vi "gfitsio-check-col-for-read.vi"(6 "row":i32, 8 "error in (no error)":errorcluster, 11 "gfits refnum":T1) -> (0 "error out":errorcluster, 3 "dup gfits refnum":T1)   [LabVIEW 2022 SP3, in "gfitsio.lvlib"]
uses:
  gfitsio.lvlib
  gfitsio-refnum.ctl
  gfitsio-error-codes.ctl
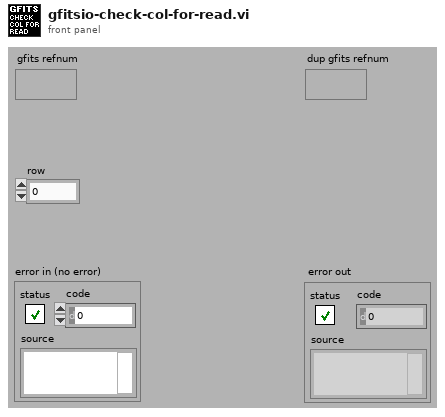
[diagram p1: front panel]
types:
  T1 = typedef "gfitsio.lvlib/gfitsio-refnum.ctl" = refnum<k1>
  T2 = typedef "gfitsio.lvlib/gfitsio-error-codes.ctl" = i32
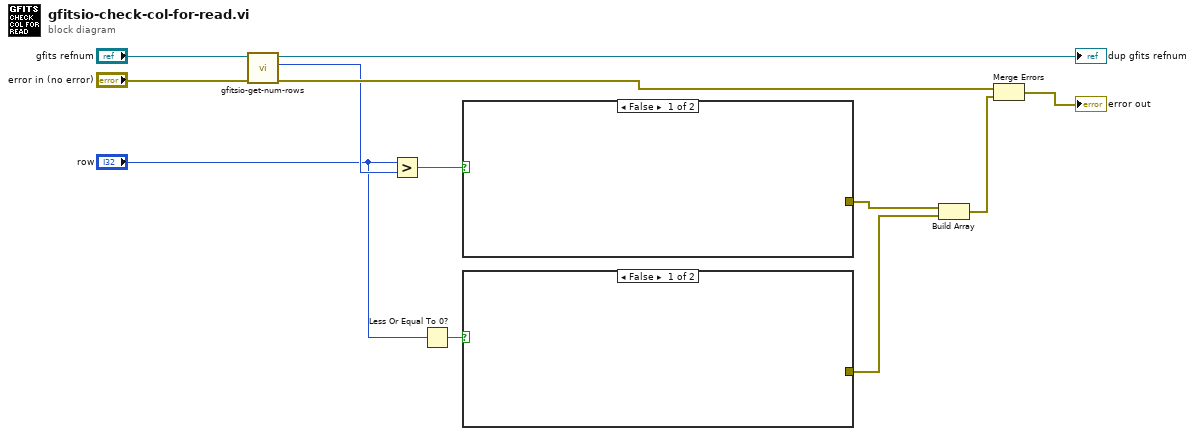
[diagram p0: block diagram]
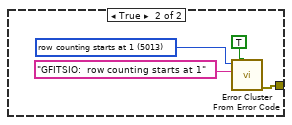
[diagram p2: hidden frame]
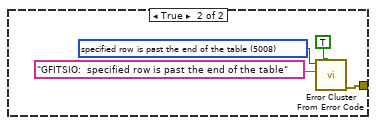
[diagram p3: hidden frame]
diagram:
  n1 = call "gfitsio-get-num-rows.vi"("error in (no error)"="error in (no error)", "gfits refnum"="gfits refnum") -> ("error out"=w11:errorcluster, "number of rows"=w9:i32, "dup gfits refnum"=→"dup gfits refnum":T1)  [unwired: 7 out]
  n2 = Greater?(x="row", y=w9) -> (0:w8:bool)
  n3 = Less Or Equal To 0?(x="row") -> (x <= 0?=w5:bool)
  n4 = case shown="False" w8 {
    tunnel: [_ w15] -> w6
    frame False {
    }
    frame True {
      w13 = T2 5008 items=["no error"=0, "dimensionality conflict"=5001, "fpixel out of image bounds"=5002, "lpixel out of image bounds"=5003, "increment size larger than image"=5004, "increment must be greater than zero"=5005, "fpixel must specify lower left corner"=5006, "named HDU not found"=5007, "specified row is past the end of the table"=5008, "wrong number of elements for column"=5009, "column is not scalar"=5010, "duplicate HDU name"=5011, "invalid table type"=5012] ("error code (0)")
      n5 = call <vilib>:"Error Cluster From Error Code.vi"("show call chain? (False)"=TRUE, "error message (\"\")"="GFITSIO:  specified row is past the end of the table" ("error message (\"\")"), "error code (0)"=w13) -> ("error out"=w15:errorcluster)  [unwired: 1 in, 5 out]
    }
  }
  n6 = case shown="False" w5 {
    tunnel: [_ w19] -> w3
    frame False {
    }
    frame True {
      w17 = T2 5013 items=["no error"=0, "dimensionality conflict"=5001, "fpixel out of image bounds"=5002, "lpixel out of image bounds"=5003, "increment size larger than image"=5004, "increment must be greater than zero"=5005, "fpixel must specify lower left corner"=5006, "named HDU not found"=5007, "specified row is past the end of the table"=5008, "wrong number of elements for column"=5009, "column is not scalar"=5010, "duplicate HDU name"=5011, "invalid table type"=5012, "row counting starts at 1"=5013] ("Ring")
      n7 = call <vilib>:"Error Cluster From Error Code.vi"("show call chain? (False)"=TRUE, "error message (\"\")"="GFITSIO:  row counting starts at 1" ("error message (\"\")"), "error code (0)"=w17) -> ("error out"=w19:errorcluster)  [unwired: 1 in, 5 out]
    }
  }
  n8 = Build Array(w6, w3) -> (w7:errorcluster[])
  n9 = Merge Errors(w11, w7) -> (→"error out":errorcluster)
